vi "Global 1.vi"() -> ()   [LabVIEW 2009]
panel:
  in  "data":string
  out "Expired":bool
  in  "count":dbl
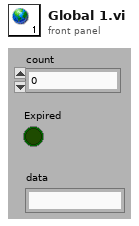
[diagram p1: front panel]
diagram:
